vi "report_generateHeader.vi"(8 "error in (no error)":errorcluster, 11 "Path in":path) -> (0 "error out":errorcluster, 3 "Path out":path)   [LabVIEW 2019]
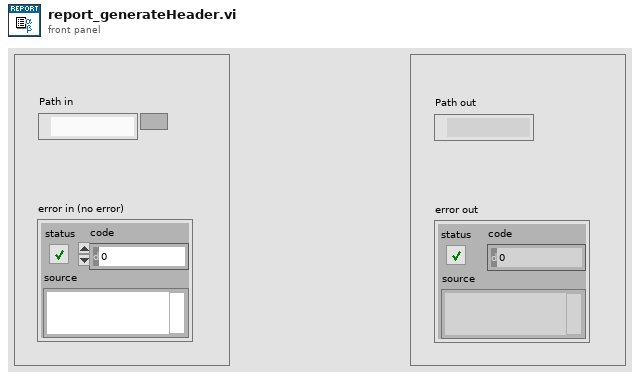
[diagram p1: front panel]
types:
  T1 = enum16{"open", "replace", "create", "open or create", "replace or create", "replace or create with confirmation"}
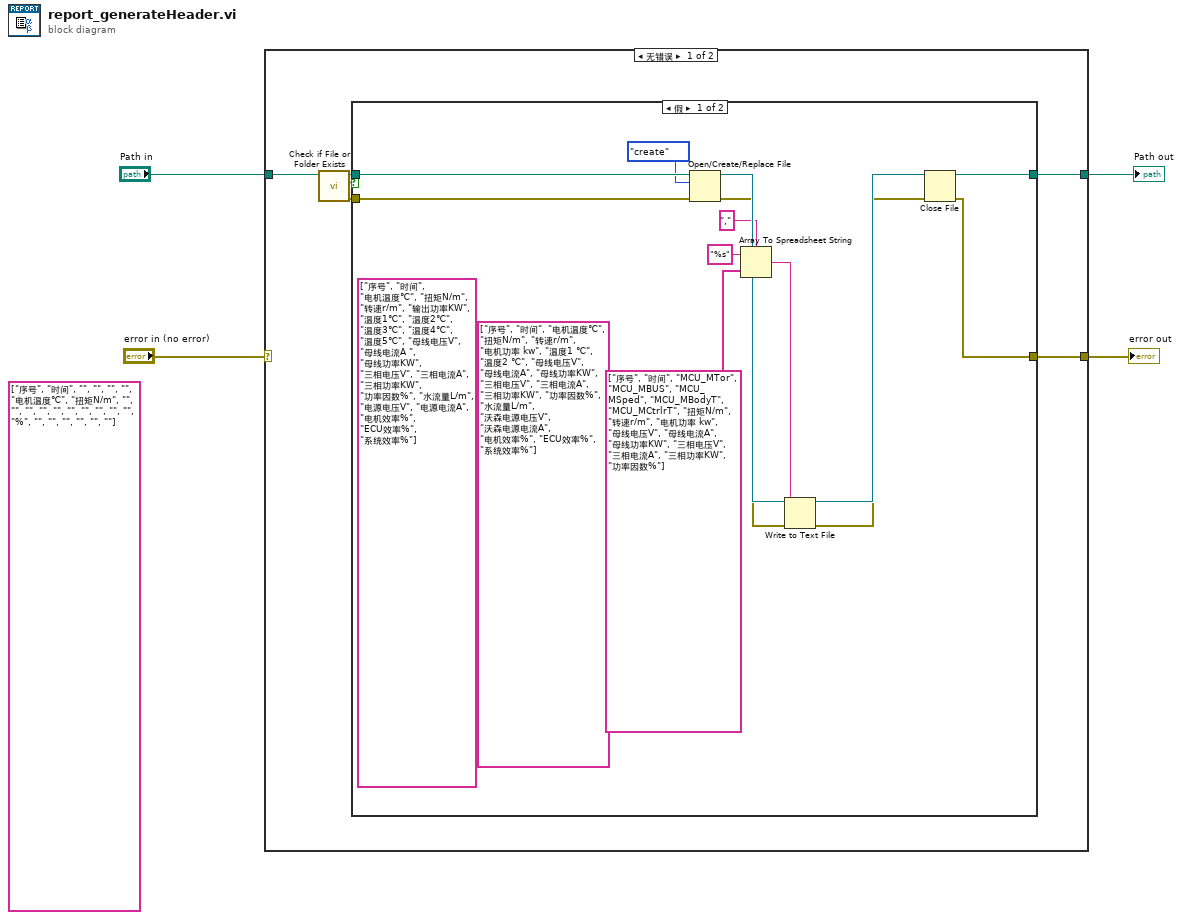
[diagram p0: block diagram]
diagram:
  (unwired) string[] ["序号", "时间", "", "", "", "", "电机温度℃", "扭矩N/m", "", "", "", "", "", "", "", "", "", "", "%", "", "", "", "", "", ""]
  n1 = case shown="无错误" "error in (no error)" {
    selector: "error in (no error)" -> [_ w27]
    tunnel: "Path in" -> [w10 w26]
    tunnel: [w7 w26] -> w3
    tunnel: [w5 w27] -> w2
    frame No Error {
      n2 = call <vilib>:"Check if File or Folder Exists.vi"("path"=w10) -> ("error out"=w6:errorcluster, "file or folder exists?"=w9:bool, "dup path"=w8:path)  [unwired: 8 in]
      n3 = case shown="假" w9 {
        tunnel: w8 -> [w23 w25]
        tunnel: [w19 w25] -> w7
        tunnel: w6 -> [w18 w24]
        tunnel: [w15 w24] -> w5
        frame False {
          (unwired) string[] ["序号", "时间", "电机温度℃", "扭矩N/m", "转速r/m", "电机功率 kw", "温度1 ℃", "温度2 ℃", "母线电压V", "母线电流A", "母线功率KW", "三相电压V", "三相电流A", "三相功率KW", "功率因数%", "水流量L/m", "沃森电源电压V", "沃森电源电流A", "电机效率%", "ECU效率%", "系统效率%"]
          (unwired) string[] ["序号", "时间", "电机温度℃", "扭矩N/m", "转速r/m", "输出功率KW", "温度1℃", "温度2℃", "温度3℃", "温度4℃", "温度5℃", "母线电压V", "母线电流A ", "母线功率KW", "三相电压V", "三相电流A", "三相功率KW", "功率因数%", "水流量L/m", "电源电压V", "电源电流A", "电机效率%", "ECU效率%", "系统效率%"]
          n4 = Open/Create/Replace File(file path (use dialog)=w23, error in=w18, operation (0:open)=T1."create") -> (refnum out=w21:refnum<file>, error out=w17:errorcluster)  [unwired: 3 in, 1 out]
          n5 = Array To Spreadsheet String(delimiter (Tab)=",", array=string[] ["序号", "时间", "MCU_MTor", "MCU_MBUS", "MCU_MSped", "MCU_MBodyT", "MCU_MCtrlrT", "扭矩N/m", "转速r/m", "电机功率 kw", "母线电压V", "母线电流A", "母线功率KW", "三相电压V", "三相电流A", "三相功率KW", "功率因数%"], 3:"%s" ("format string")) -> (spreadsheet string=w12:string)
          n6 = Write to Text File(file (use dialog)=w21, text=w12, error in=w17) -> (refnum out=w20:refnum<file>, error out=w16:errorcluster)  [unwired: 1 in, 1 out]
          n7 = Close File(refnum=w20, error in=w16) -> (path=w19:path, error out=w15:errorcluster)
        }
        frame True {
        }
      }
    }
    frame Error {
    }
  }
  "Path out" <- w3
  "error out" <- w2
